vi "Test Inversor API.vi"() -> ()   [LabVIEW 2019]
doc: "Inversor API Tester."
uses:
  <vilib>/Utility/error.llb/DialogType.ctl
  Inversor.lvlib
panel:
  in  "Numeric":dbl
  in  "Request Simple":bool
  out "Command":string
  in  "Voltage":dbl
  in  "Set Voltage":bool
  out "Module ID":i32
  in  "Combo Box":string(combo)
  out "Map":map{i32, string}(c390)
  in  "Nombre":string
  out "last error":errorcluster
  in  "Show Diagram on Init":bool
  in  "Run as Singleton?":bool
  in  "Show Block Diagram":bool
  in  "Refresh Modules":bool
  out "Active Modules":string[](array[string])
  in  "Stop Module":bool
  in  "Select Module":i32(ring)=-1 caption="Select Module\nTo send Request to" items=["All"=-1, "1"=1, "2"=2, "3"=3, "4"=4]
  in  "Run New Module":bool
  in  "Hide Module Panel":bool
  in  "Show Module Panel":bool
  out "Status":string
  # "This VI tests the API for the Module."
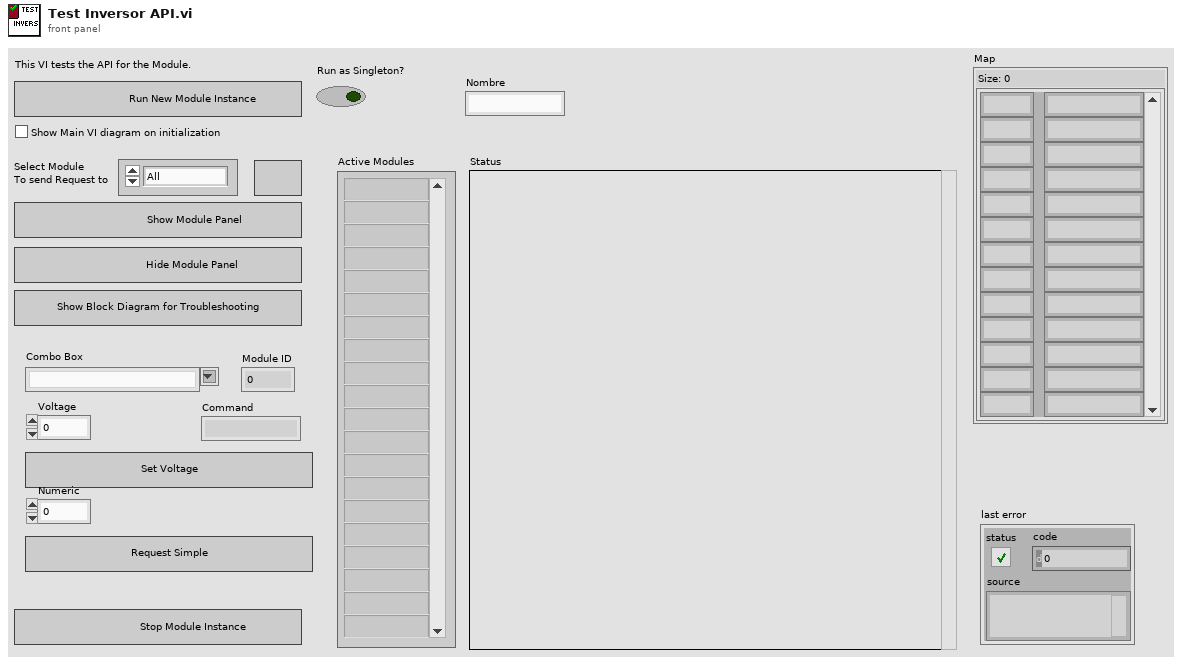
[diagram p1: front panel]
types:
  T1 = typedef "Inversor.lvlib/Broadcast Events--cluster.ctl" = cluster{"Module Did Init":refnum<user-event>, "Status Updated":refnum<user-event>, "Error Reported":refnum<user-event>, "Module Did Stop":refnum<user-event>, "Update Module Execution Status":refnum<user-event>}
  T2 = typedef "DialogType.ctl" = u16
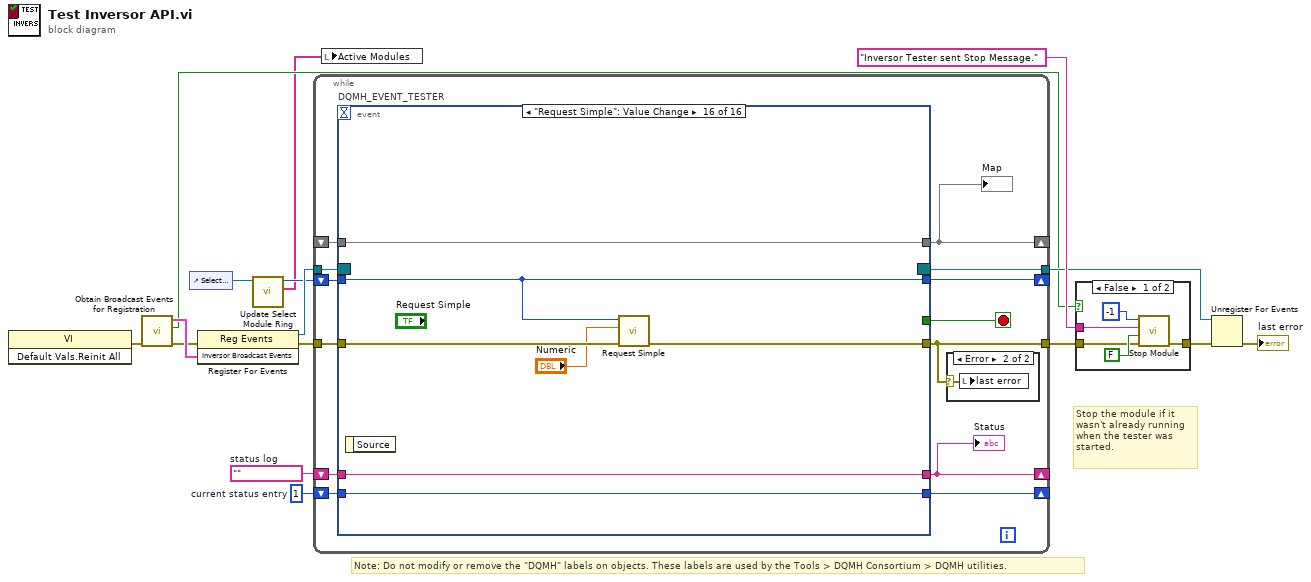
[diagram p0: block diagram]
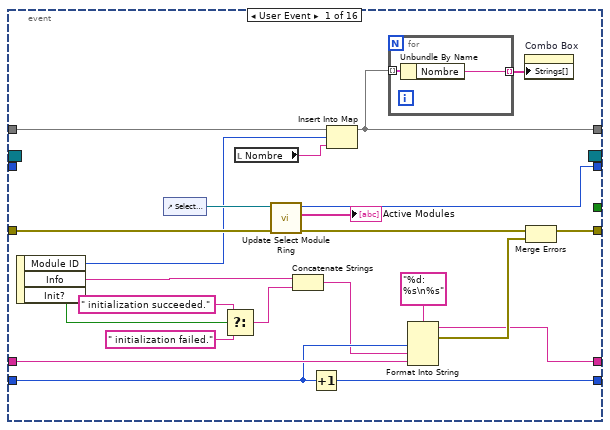
[diagram p4: hidden frame]
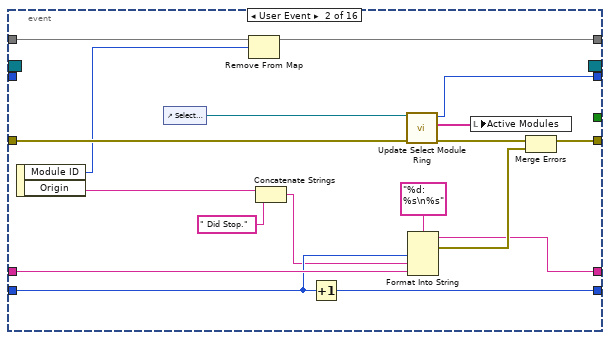
[diagram p5: hidden frame]
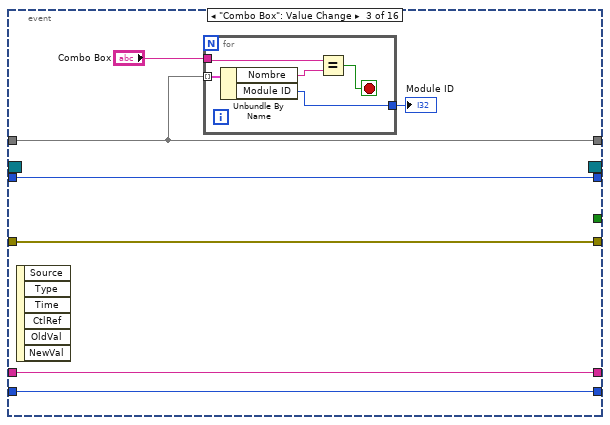
[diagram p6: hidden frame]
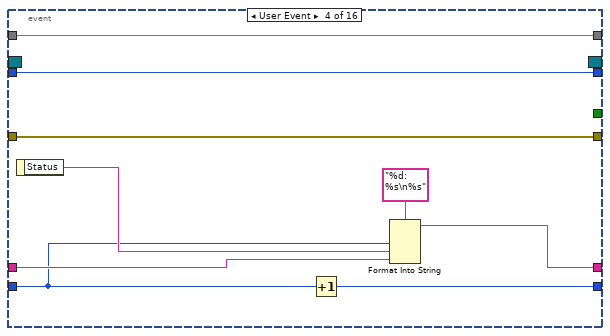
[diagram p7: hidden frame]
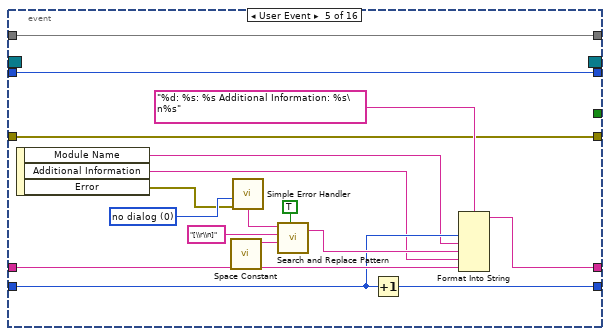
[diagram p8: hidden frame]
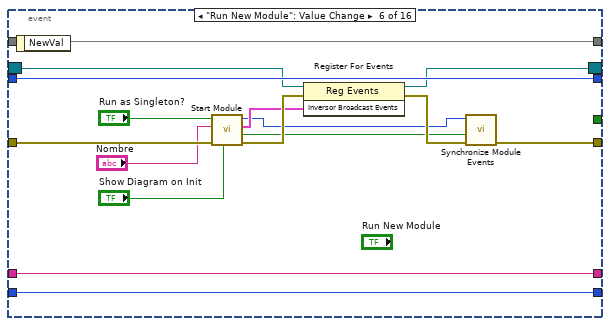
[diagram p9: hidden frame]
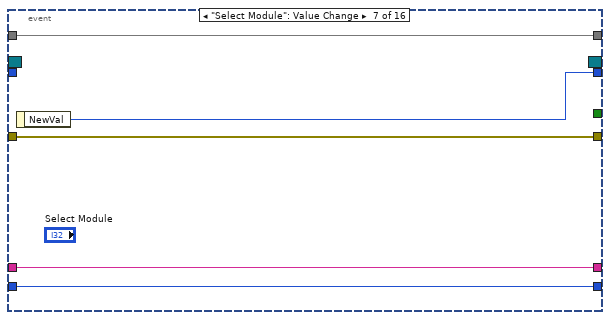
[diagram p10: hidden frame]
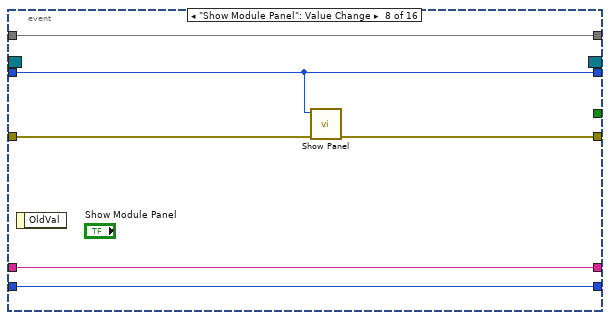
[diagram p11: hidden frame]
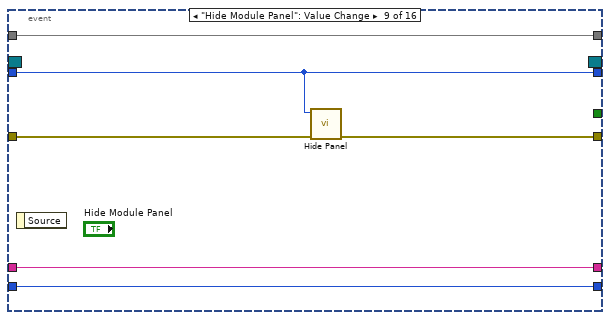
[diagram p12: hidden frame]
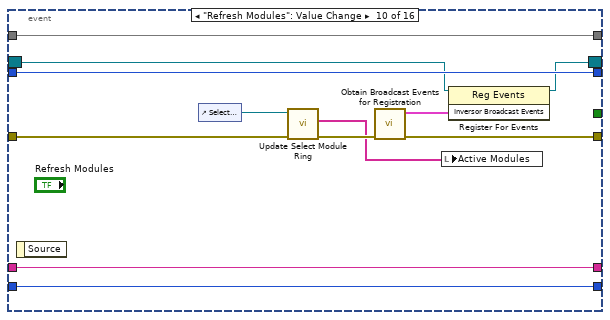
[diagram p13: hidden frame]
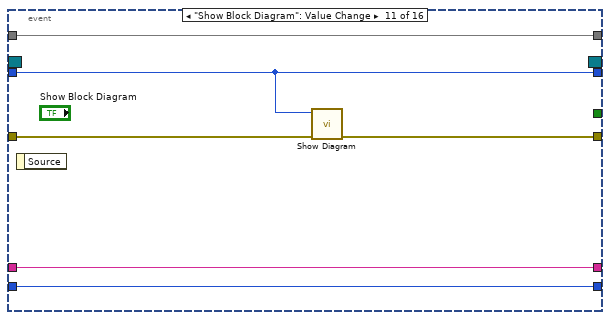
[diagram p14: hidden frame]
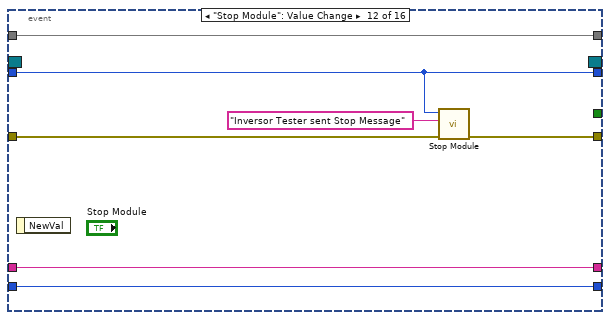
[diagram p15: hidden frame]
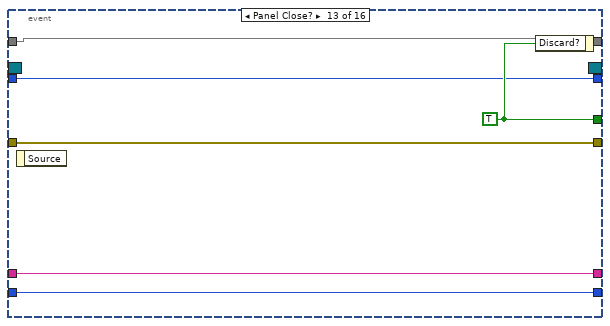
[diagram p16: hidden frame]
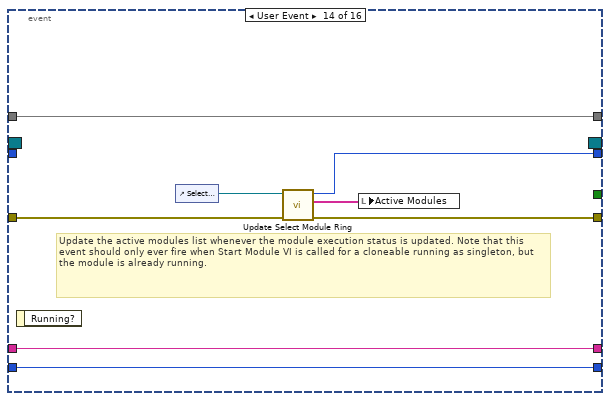
[diagram p17: hidden frame]
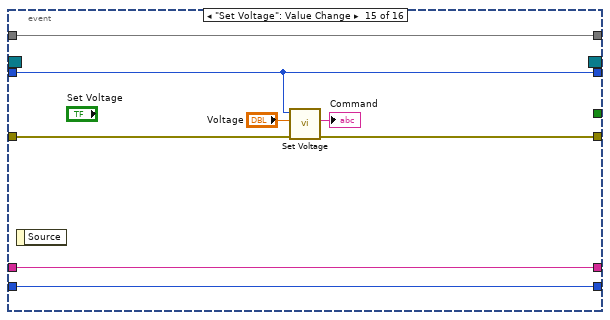
[diagram p18: hidden frame]
diagram:
  w13 = 1  # current status entry
  w14 = ""  # status log
  # "Stop the module if it wasn't already running when the tester was started."
  # "Note: Do not modify or remove the \"DQMH\" labels on objects. These labels are used by the Tools > DQMH Consortium > DQMH utilities."
  n1 = invoke class="VI" method="Default Vals.Reinit All"() -> (error out=w8:errorcluster)  [unwired: 3 in, 2 out]
  n2 = call "Obtain Broadcast Events for Registration.vi"("error in"=w8) -> ("error out"=w7:errorcluster, "Already running?"=w6:bool, "Inversor Broadcast Events"=w12:T1)  [unwired: 8 in]
  n3 = control-ref of="Select Module"() -> (w3:refnum<vi>)
  n4 = register-events(error in=w7, w12) -> (reference out=w16:refnum<event-registration>, error out=w11:errorcluster)  [unwired: 1 in]
  n5 = call "Update Select Module Ring.vi"("Select Module Ring Ref"=w3) -> ("Active Modules (Array)"=w1:string[], "New Module Ring Value"=w2:i32)  [unwired: 8 in, 1 out]
  n6 = while {
    tunnel: w16 -> [w29]
    tunnel: [w20] -> w5
    tunnel: w11 -> [w28]
    shift-right: [w24] -> _
    shift-left: w14 -> [w26]
    shift-right: [w25] -> _
    shift-left: w13 -> [w27]
    shift-right: [w22] -> _
    shift-left: w2 -> [w23]
    tunnel: [w21] -> w9
    shift-right: [w18] -> _
    shift-left: _ -> [w17]
    stop <- w19 stop-if-true
    n7 = event "DQMH_EVENT_TESTER" shown="[15] \"Request Simple\": Value Change" {
      selector: w29 -> [_ _ _ _ _ w121 _ _ _ w151 _ _ _ _ _ _]
      dyn-events: [_ _ _ _ _ w120 _ _ _ w150 _ _ _ _ _ _] -> w21
      timeout: _ -> [_ _ _ _ _ _ _ _ _ _ _ _ _ _ _ _]
      tunnel: [_ _ _ _ _ _ _ _ _ _ _ _ w175 _ _ _] -> w19
      tunnel: [w43 w65 w80 w94 w99 w119 w132 w137 w143 w147 w159 w165 w174 w179 w186 w193] -> w20
      tunnel: w28 -> [w45 w67 w80 w94 w99 w122 w132 w138 w144 w152 w162 w166 w174 w180 w191 w198]
      tunnel: w27 -> [w50 w70 w78 w87 w102 w124 w130 w135 w141 w155 w160 w168 w172 w182 w189 w196]
      tunnel: w26 -> [w51 w71 w79 w90 w103 w125 w131 w136 w142 w156 w161 w169 w173 w183 w190 w197]
      tunnel: [w48 w68 w79 w91 w101 w125 w131 w136 w142 w156 w161 w169 w173 w183 w190 w197] -> w24
      tunnel: [w49 w69 w78 w93 w100 w124 w130 w135 w141 w155 w160 w168 w172 w182 w189 w196] -> w25
      tunnel: w23 -> [_ _ w77 w88 w111 w123 _ w134 w140 w154 w158 w167 w171 _ w188 w195]
      tunnel: [w40 w62 w77 w88 w111 w123 w129 w134 w140 w154 w158 w167 w171 w178 w188 w195] -> w22
      tunnel: [w32 w56 w76 w86 w95 w112 w128 w133 w139 w145 w157 w163 w170 w176 w187 w194] -> w18
      tunnel: w17 -> [w33 w57 w76 w86 w95 w112 w128 w133 w139 w145 w157 w163 w170 w176 w187 w194]
      event User Event {
        n8 = event-data() -> ("Module ID"=w35:i32, "Info"=w47:string, "Init?"=w37:bool)  [unwired: 1 in]
        n9 = control-ref of="Select Module"() -> (w42:refnum<vi>)
        n10 = Select(t=" initialization succeeded.", s=w37, f=" initialization failed.") -> (s? t:f=w36:string)
        n11 = local read "Nombre"() -> (w34:string)
        n12 = call "Update Select Module Ring.vi"("error in"=w45, "Select Module Ring Ref"=w42) -> ("error out"=w44:errorcluster, "Active Modules (Array)"=→"Active Modules":string[], "New Module Ring Value"=w40:i32)  [unwired: 7 in]
        n13 = Concatenate Strings(w47, w36) -> (w46:string)
        n14 = Increment(x=w50) -> (x+1=w49:i32)
        n15 = Insert Into Map(map in=w33, key=w35, value=w34) -> (map out=w32:map{i32, string})  [unwired: 2 out]
        n16 = for {
          tunnel: w32 -> [w55] mode=indexing
          tunnel: [w54] -> w31 mode=indexing
          n17 = Unbundle By Name(w55) -> ("Nombre"=w54:string)
        }
        n18 = Format Into String(format string="%d: %s\n%s", w50, w46, w51) -> (resulting string=w48:string, error out=w53:errorcluster)  [unwired: 2 in]
        n19 = property on="Combo Box" class="CmbBox"("Strings[]"=w31) -> ()  [unwired: 2 in, 2 out]
        n20 = Merge Errors(w44, w53) -> (w43:errorcluster)
      }
      event User Event {
        n21 = event-data() -> ("Module ID"=w58:i32, "Origin"=w60:string)  [unwired: 1 in]
        n22 = control-ref of="Select Module"() -> (w64:refnum<vi>)
        n23 = Remove From Map(10:w58, 11:w57) -> (3:w56:map{i32, string})  [unwired: 2 out]
        n24 = Concatenate Strings(w60, " Did Stop.") -> (w59:string)
        n25 = Increment(x=w70) -> (x+1=w69:i32)
        n26 = call "Update Select Module Ring.vi"("error in"=w67, "Select Module Ring Ref"=w64) -> ("error out"=w66:errorcluster, "Active Modules (Array)"=w63:string[], "New Module Ring Value"=w62:i32)  [unwired: 7 in]
        n27 = Format Into String(format string="%d: %s\n%s", w70, w59, w71) -> (resulting string=w68:string, error out=w73:errorcluster)  [unwired: 2 in]
        n28 = local write "Active Modules"(w63) -> ()
        n29 = Merge Errors(w66, w73) -> (w65:errorcluster)
      }
      event "Combo Box": Value Change {
        n30 = event-data() -> ()  [unwired: 1 in, 6 out]
        n31 = for {
          tunnel: w76 -> [w85] mode=indexing
          tunnel: "Combo Box" -> [w82]
          tunnel: [w81] -> w74
          stop <- w84 stop-if-true
          n32 = Unbundle By Name(w85) -> ("Nombre"=w83:string, "Module ID"=w81:i32)
          n33 = Equal?(x=w82, y=w83) -> (x = y?=w84:bool)
        }
        "Module ID" <- w74
      }
      event User Event {
        n34 = event-data() -> ("Status"=w89:string)  [unwired: 1 in]
        n35 = Increment(x=w87) -> (x+1=w93:i32)
        n36 = Format Into String(format string="%d: %s\n%s", w87, w89, w90) -> (resulting string=w91:string)  [unwired: 2 in, 1 out]
      }
      event User Event {
        w104 = T2 0 items=["no dialog", "OK message", "continue or stop message", "OK message + warnings", "continue/stop + warnings"] ("type of dialog (OK msg:1)")
        n37 = event-data() -> ("Module Name"=w98:string, "Additional Information"=w97:string, "Error"=w96:errorcluster)  [unwired: 1 in]
        n38 = call <vilib>:"Space Constant.vi"() -> ("String"=w108:string)
        n39 = call <vilib>:"Simple Error Handler.vi"("type of dialog (OK msg:1)"=w104, "error in (no error)"=w96) -> ("message"=w105:string)  [unwired: 3 in, 4 out]
        n40 = call <vilib>:"Search and Replace Pattern.vi"("string"=w105, "regular expression (\"\")"="[\\r\\n]" ("regular expression (\"\")"), "replace string (\"\")"=w108, "replace all? (F)"=TRUE ("replace all CR/LF with spaces")) -> ("result string"=w106:string)  [unwired: 1 in, 1 out]
        n41 = Increment(x=w102) -> (x+1=w100:i32)
        n42 = Format Into String(format string="%d: %s: %s Additional Information: %s\n%s", w102, w98, w106, w97, w103) -> (resulting string=w101:string)  [unwired: 2 in, 1 out]
      }
      event "Run New Module": Value Change {
        n43 = event-data() -> ()  [unwired: 1 in, 1 out]
        n44 = call "Start Module.vi"("Show Main VI Diagram on Init (F)"="Show Diagram on Init", "error in"=w122, "Nombre"="Nombre", "Run as Singleton? (F)"="Run as Singleton?") -> ("error out"=w126:errorcluster, "Wait for Event Sync?"=w118:bool, "Inversor Broadcast Events"=w117:T1, "Module ID"=w114:i32)  [unwired: 3 in, 1 out]
        n45 = register-events(reference=w121, error in=w126, w117) -> (reference out=w120:refnum<event-registration>, error out=w127:errorcluster)
        n46 = call "Synchronize Module Events.vi"("error in"=w127, "Wait for Event Sync?"=w118, "Module ID in"=w114) -> ("error out"=w119:errorcluster)  [unwired: 7 in, 1 out]
      }
      event "Select Module": Value Change {
        n47 = event-data() -> ("NewVal"=w129:i32)  [unwired: 1 in]
      }
      event "Show Module Panel": Value Change {
        n48 = event-data() -> ()  [unwired: 1 in, 1 out]
        n49 = call "Show Panel.vi"("error in"=w138, "Module ID"=w134) -> ("error out"=w137:errorcluster)  [unwired: 9 in]
      }
      event "Hide Module Panel": Value Change {
        n50 = event-data() -> ()  [unwired: 1 in, 1 out]
        n51 = call "Hide Panel.vi"("error in"=w144, "Module ID"=w140) -> ("error out"=w143:errorcluster)  [unwired: 9 in]
      }
      event "Refresh Modules": Value Change {
        n52 = event-data() -> ()  [unwired: 1 in, 1 out]
        n53 = control-ref of="Select Module"() -> (w153:refnum<vi>)
        n54 = call "Update Select Module Ring.vi"("error in"=w152, "Select Module Ring Ref"=w153) -> ("error out"=w148:errorcluster, "Active Modules (Array)"=w146:string[])  [unwired: 7 in, 1 out]
        n55 = call "Obtain Broadcast Events for Registration.vi"("error in"=w148) -> ("error out"=w147:errorcluster, "Inversor Broadcast Events"=w149:T1)  [unwired: 8 in, 1 out]
        n56 = local write "Active Modules"(w146) -> ()
        n57 = register-events(reference=w151, w149) -> (reference out=w150:refnum<event-registration>)  [unwired: 1 in, 1 out]
      }
      event "Show Block Diagram": Value Change {
        n58 = event-data() -> ()  [unwired: 1 in, 1 out]
        n59 = call "Show Diagram.vi"("error in"=w162, "Module ID"=w158) -> ("error out"=w159:errorcluster)  [unwired: 9 in]
      }
      event "Stop Module": Value Change {
        n60 = event-data() -> ()  [unwired: 1 in, 1 out]
        n61 = call "Stop Module.vi"("error in"=w166, "Origin"="Inversor Tester sent Stop Message", "Module ID"=w167) -> ("error out"=w165:errorcluster)  [unwired: 8 in]
      }
      event Panel Close? {
        w175 = TRUE ("Discard?")
        n62 = event-data() -> ()  [unwired: 1 in, 1 out]
        n63 = event-data("Discard?"=w175) -> ()  [unwired: 1 in, 1 out]
      }
      event User Event {
        # "Update the active modules list whenever the module execution status is updated. Note that this event should only ever fire when Start Module VI is called for a cloneable running as singleton, but the module is already running."
        n64 = event-data() -> ()  [unwired: 1 in, 1 out]
        n65 = control-ref of="Select Module"() -> (w181:refnum<vi>)
        n66 = call "Update Select Module Ring.vi"("error in"=w180, "Select Module Ring Ref"=w181) -> ("error out"=w179:errorcluster, "Active Modules (Array)"=w177:string[], "New Module Ring Value"=w178:i32)  [unwired: 7 in]
        n67 = local write "Active Modules"(w177) -> ()
      }
      event "Set Voltage": Value Change {
        n68 = event-data() -> ()  [unwired: 1 in, 1 out]
        n69 = call "Set Voltage.vi"("error in"=w191, "Voltage"="Voltage", "Module ID"=w188) -> ("error out"=w186:errorcluster, "Command"=→"Command":string)  [unwired: 6 in, 1 out]
      }
      event "Request Simple": Value Change {
        n70 = event-data() -> ()  [unwired: 1 in, 1 out]
        n71 = call "Request Simple.vi"("error in"=w198, "Numeric"="Numeric", "Module ID"=w195) -> ("error out"=w193:errorcluster)  [unwired: 8 in]
      }
    }
    "Status" <- w24
    "Map" <- w18
    n72 = case shown="Error" w20 {
      selector: w20 -> [_ w30]
      frame No Error {
      }
      frame Error {
        n73 = local write "last error"(w30) -> ()
      }
    }
  }
  n74 = local write "Active Modules"(w1) -> ()
  n75 = case shown="False" w6 {
    tunnel: [w203 w204] -> w15
    tunnel: "Inversor Tester sent Stop Message." ("Origin") -> [w202 _]
    tunnel: w5 -> [w199 w204]
    frame False {
      n76 = call "Stop Module.vi"("error in"=w199, "Wait for Module to stop? (F)"=FALSE ("Wait for Module to stop?"), "Origin"=w202, "Module ID"=-1 ("Stop all")) -> ("error out"=w203:errorcluster)  [unwired: 7 in]
    }
    frame True {
    }
  }
  n77 = Unregister For Events(event registration refnum=w9, error in=w15) -> (error out=→"last error":errorcluster)
